vi "viReadSerialExtractFrame.vi"(0 "VISA resource name in":refnum<visa-resource-name>, 1 "error in (no error)":errorcluster) -> (2 "VISA resource name out":refnum<visa-resource-name>, 3 "Data":dbl[](array[numeric]), 4 "error out":errorcluster)   [LabVIEW 2009]
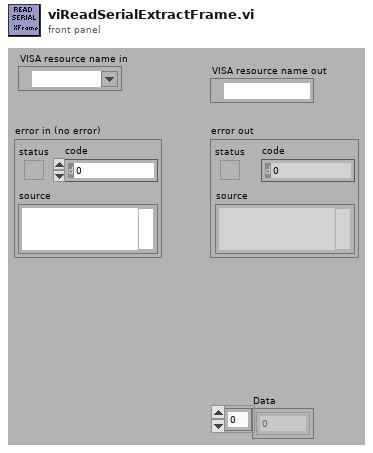
[diagram p1: front panel]
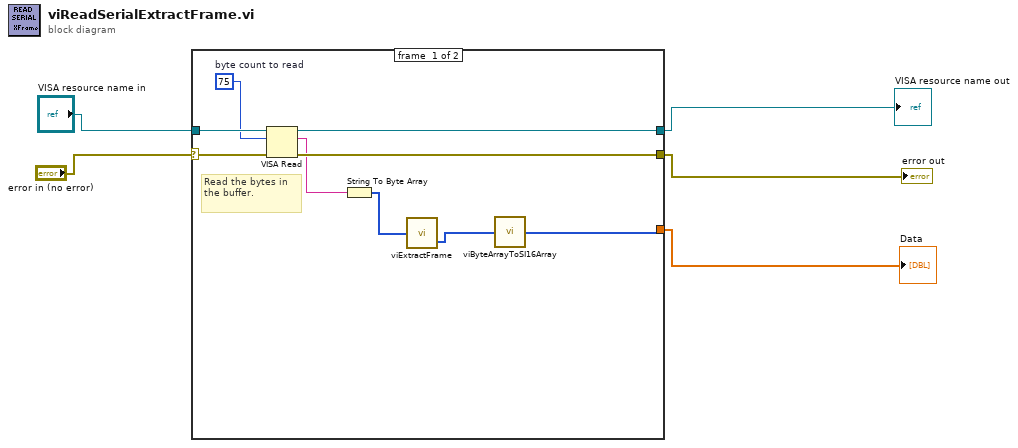
[diagram p0: block diagram]
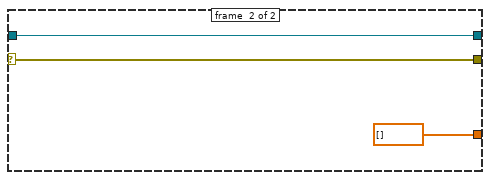
[diagram p2: hidden frame]
diagram:
  n1 = case "Read bytes from port." shown="No Error" "error in (no error)" {
    selector: "error in (no error)" -> [w11 w16]
    tunnel: [w13 w16] -> w1
    tunnel: [w14 w17] -> w5
    tunnel: "VISA resource name in" -> [w12 w17]
    tunnel: [w8 dbl[] [] ("Array 2")] -> w4
    frame #0 {
      w10 = u32 75  # byte count to read
      # "Read the bytes in the buffer."
      n2 = VISA Read(VISA resource name=w12, byte count=w10, error in (no error)=w11) -> (VISA resource name out=w14:refnum<visa-resource-name>, read buffer=w7:string, error out=w13:errorcluster)  [unwired: 1 out]
      n3 = String To Byte Array(string=w7) -> (unsigned byte array=w6:u8[])
      n4 = call "viExtractFrame.vi"("input variable"=w6) -> ("output variable"=w9:u8[])  [unwired: 1 out]
      n5 = call "viByteArrayToSI16Array.vi"("input variable"=w9) -> ("output variable"=w8:i16[])
    }
    frame #1 {
      # "Error occurred \nreading Bytes at \nSerial Port"
    }
  }
  "error out" <- w1
  "VISA resource name out" <- w5
  "Data" <- w4
